vi "FTW-Endpoint-Destroy.vi"(0 "FTW ØMQ Endpoint":refnum<class "FTW-Endpoint-ZMQ.lvclass">, 5 "Force Destroy":bool, 11 "error in":errorcluster) -> (15 "error out":errorcluster)   [LabVIEW 2012, in "FTW-Endpoint-ZMQ.lvclass"]
uses:
  FTW-Endpoint-ZMQ.lvclass
  FTW-Endpoint-ZMQ.lvclass/FTW-Endpoint-ZMQ.ctl
panel:
  # "Inputs"
  # "Outputs"
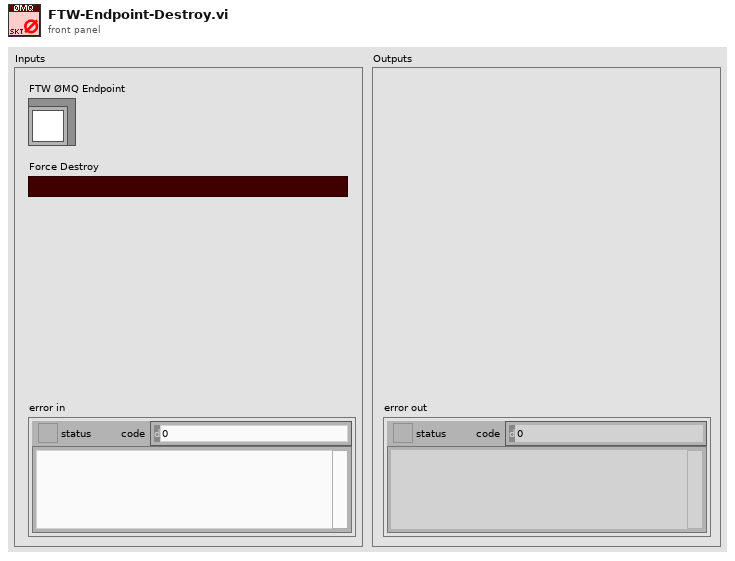
[diagram p1: front panel]
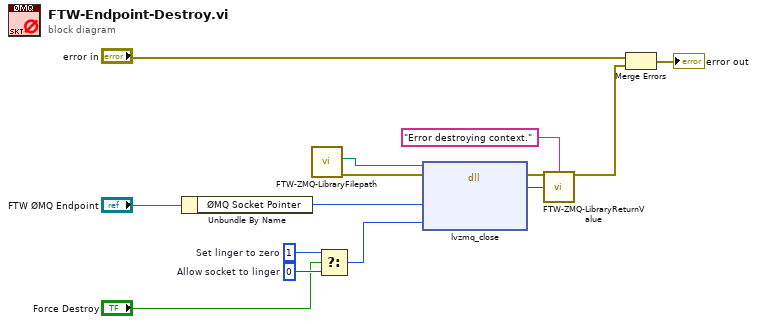
[diagram p0: block diagram]
diagram:
  w8 = 1  # Set linger to zero
  w7 = 0  # Allow socket to linger
  n1 = Unbundle By Name("FTW ØMQ Endpoint") -> ("ØMQ Socket Pointer"=w1:u64)
  n2 = call "FTW-ZMQ-LibraryFilepath.vi"() -> ("error out"=w10:errorcluster, "FTW-ZMQ Library Filepath"=w9:path)  [unwired: 9 in, 1 out]
  n3 = Select(t=w8, s="Force Destroy", f=w7) -> (s? t:f=w6:i32)
  n4 = dll-call lib="?" fn="lvzmq_close" ("libzmq.dll:zmq_close")(path in=w9, error in=w10, "Socket Pointer"=w1, "Flags"=w6) -> (error out=w3:errorcluster, "Return Value"=w4:i32)  [unwired: 3 in, 1 out]
  n5 = call "FTW-ZMQ-LibraryReturnValue.vi"("error in"=w3, "Error Message"="Error destroying context.", "Return Value"=w4) -> ("error out"=w11:errorcluster)  [unwired: 12 in]
  n6 = Merge Errors("error in", w11) -> (→"error out":errorcluster)
